vi "GetParam.vi"(8 "error in (no error)":errorcluster caption="entrée d'erreur (pas d'erreur)", 11 "Argmin.lvclass":refnum<class "Argmin.lvclass">) -> (0 "error out":errorcluster caption="sortie d'erreur", 2 "pairwise_distances_argmin":T1={"axis"=1, "metric "="euclidean", "metric_kwargs"={"metric"=[], "kwargs"=[]}}, 3 "Argmin.lvclass":refnum<class "Argmin.lvclass">)   [LabVIEW 2020, in "Argmin.lvclass"]
doc: "Get Parameters"
uses:
  Argmin.lvclass
  Argmin.lvclass/Argmin.ctl
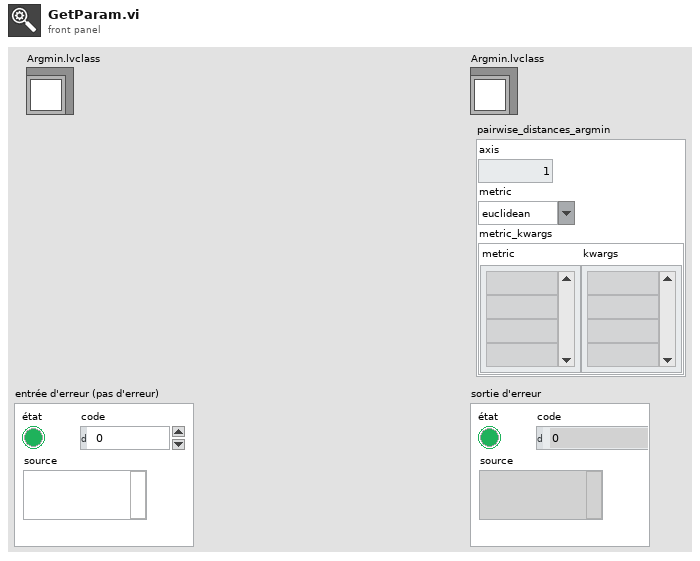
[diagram p1: front panel]
types:
  T1 = cluster{"axis":i32, "metric ":string, "metric_kwargs":cluster{"metric":string[], "kwargs":string[]}}
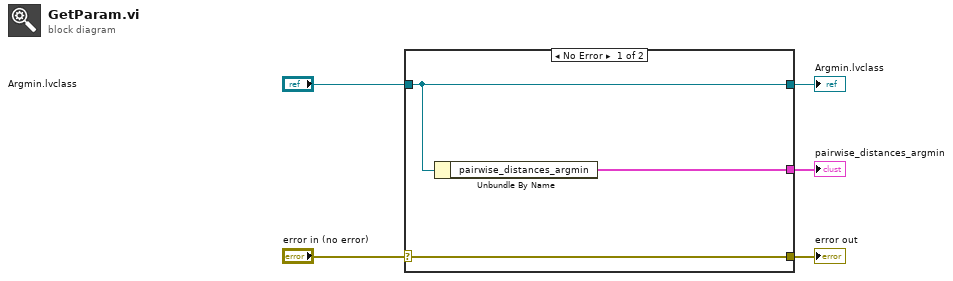
[diagram p0: block diagram]
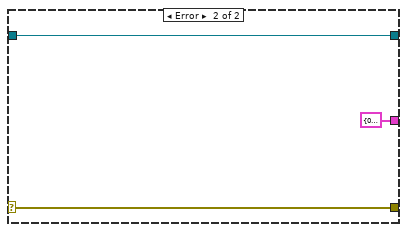
[diagram p2: hidden frame]
diagram:
  n1 = case shown="No Error" "error in (no error)" {
    selector: "error in (no error)" -> [w8 w10]
    tunnel: [w8 w10] -> w4
    tunnel: [w7 w11] -> w2
    tunnel: "Argmin.lvclass" -> [w7 w11]
    tunnel: [w6 T1 {"axis"=0, "metric "="", "metric_kwargs"={"metric"=[], "kwargs"=[]}} ("pairwise_distances_argmin")] -> w1
    frame No Error {
      n2 = Unbundle By Name(w7) -> ("pairwise_distances_argmin"=w6:T1)
    }
    frame Error {
    }
  }
  "error out" <- w4
  "Argmin.lvclass" <- w2
  "pairwise_distances_argmin" <- w1
